vi "Interface.vi"() -> ()   [LabVIEW 2016, in "Command Interface.lvclass"]
uses:
  Command Interface.lvclass
  Universal Robot/Universal Robot.lvclass
  C:/_Code/Development/UR Dashboard Server/Classes/Application Interface/Application Interface.lvclass
  Application/Application.lvclass
  Application Interface/Application Interface.lvclass
panel:
  in  "command":u16(ring) items=["Load", "Play", "Stop", "Pause", "Quit", "Shutdown", "Running", "Robotmode", "get loaded program", "popup", "close popup", "addToLog", "IsProgramSaved", "programState", "PolyscopeVersion", "set operational mode", "clear operational mode", "power on", "power off", "brake release", "safetymode", "safetystatus", "unlock protective stop", "close safety popup", "load installation", "restart safety", "get operational mode", "is in remote control", "get serial number", "get robot model", "generate flight report", "generate support file"]
  in  "input":string
  out "inputType":string
  out "warning":string
  in  "send":bool
  out "returnStatus":string
  out "data":string
  in  "interface":refnum<class "Command Interface.lvclass">
  in  "robot":refnum<class "Universal Robot.lvclass">
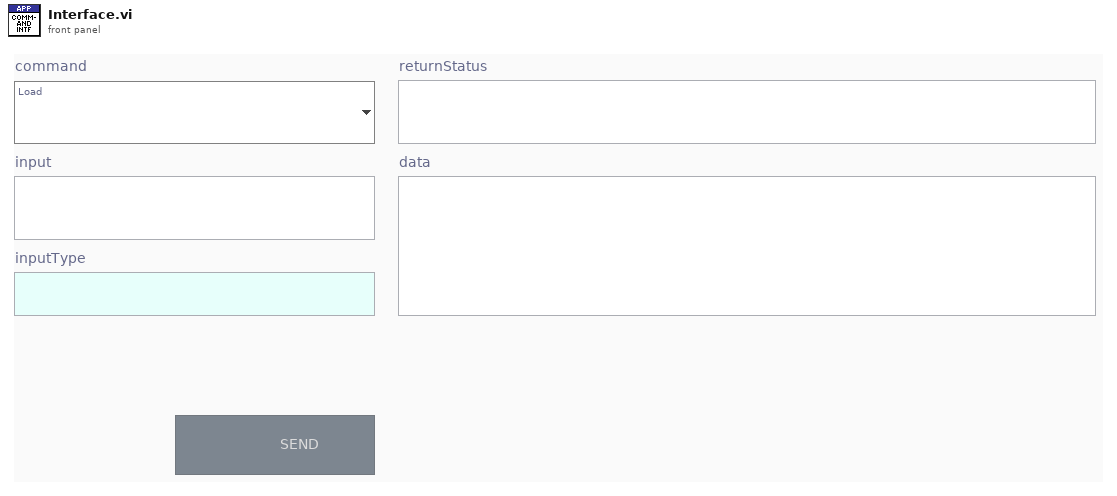
[diagram p1: front panel]
types:
  T1 = enum8{"Enabled", "Disabled", "Disabled and Grayed Out"}
  T2 = typedef "Application.lvclass/FrontPanelControls.ctl" = cluster{"General Interface":refnum<vi>, "Program Interface":refnum<vi>, "Command Interface":refnum<vi>}
  T3 = typedef "Universal Robot.lvclass/PolyScopeCommand.ctl" = cluster{"Command":string, "Input":bool, "Input Type":string, "Remote Mode Required":bool, "Min Version":T4, "Deprecated":bool}
  T4 = typedef "Universal Robot.lvclass/PolyScopeVersion.ctl" = cluster{"Major":i32, "Minor":i32, "Fix":i32, "Build":i32}
  T5 = typedef "Universal Robot.lvclass/RobotStatus.ctl" = cluster{"Robot Mode":T6, "Operational Mode":T7, "Safety Status":T8, "Remote Control":bool}
  T6 = typedef "Universal Robot.lvclass/RobotMode.ctl" = enum16{"INVALID", "NO_CONTROLLER", "DISCONNECTED", "CONFIRM_SAFETY", "BOOTING", "POWER_OFF", "POWER_ON", "IDLE", "BACKDRIVE", "RUNNING"}
  T7 = typedef "Universal Robot.lvclass/OperationalMode.ctl" = enum16{"NONE", "MANUAL", "AUTOMATIC"}
  T8 = typedef "Universal Robot.lvclass/SafetyStatus.ctl" = enum16{"INVALID", "NORMAL", "REDUCED", "PROTECTIVE_STOP", "RECOVERY", "SAFEGAURD_STOP", "SYSTEM_EMERGENCY_STOP", "ROBOT_EMERGENCY_STOP", "VIOLATION", "FAULT", "AUTOMATIC_MODE_SAFEGAURD_STOP", "SYSTEM_THREE_POSITION_ENABLING_STOP"}
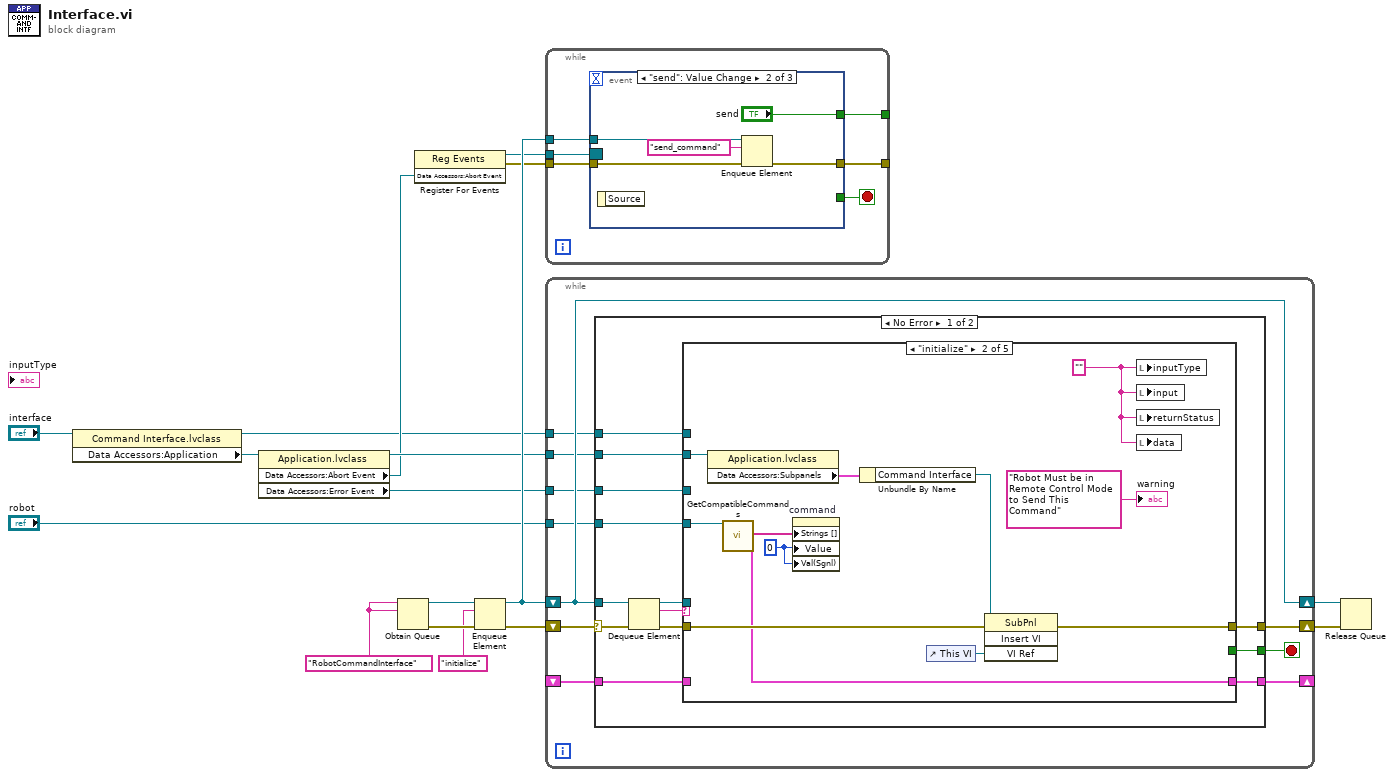
[diagram p0: block diagram]
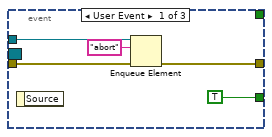
[diagram p2: hidden frame]
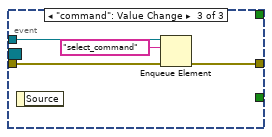
[diagram p3: hidden frame]
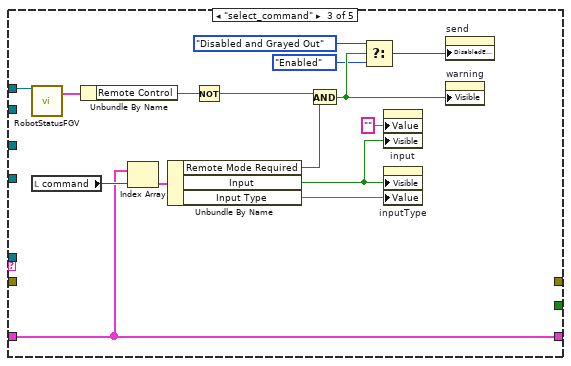
[diagram p5: hidden frame]
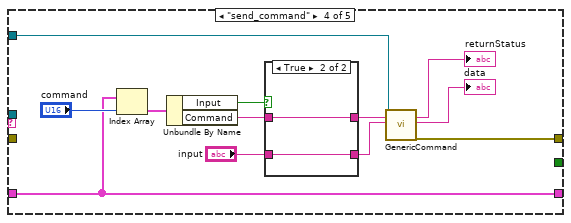
[diagram p6: hidden frame]
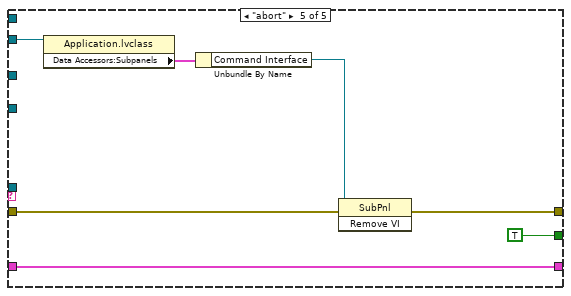
[diagram p8: hidden frame]
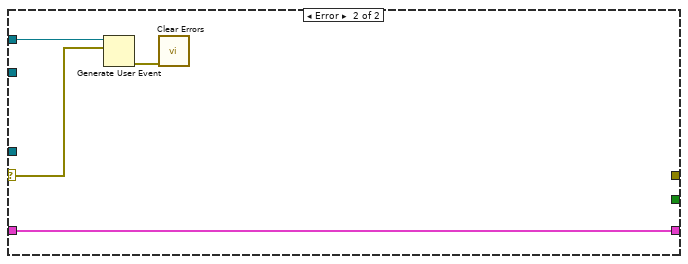
[diagram p9: hidden frame]
diagram:
  w12 = "RobotCommandInterface" ("name (unnamed)")
  n1 = property class="Command Interface.lvclass"(reference="interface") -> (reference out=w1:refnum<class "Command Interface.lvclass">, "Data Accessors:Application"=w6:refnum<class "Application.lvclass">)  [unwired: 1 in, 1 out]
  n2 = property class="Application.lvclass"(reference=w6) -> (reference out=w5:refnum<class "Application.lvclass">, "Data Accessors:Abort Event"=w4:refnum<user-event>, "Data Accessors:Error Event"=w3:refnum<user-event>)  [unwired: 1 in, 1 out]
  n3 = Obtain Queue(name (unnamed)=w12, element data type=w12) -> (queue out=w16:refnum<queue>, error out=w17:errorcluster)  [unwired: 3 in, 1 out]
  n4 = register-events(w4) -> (reference out=w8:refnum<event-registration>, error out=w9:errorcluster)  [unwired: 2 in]
  n5 = Enqueue Element(queue=w16, element="initialize", error in (no error)=w17) -> (queue out=w13:refnum<queue>, error out=w14:errorcluster)  [unwired: 1 in, 1 out]
  n6 = while {
    tunnel: w13 -> [w23]
    tunnel: w9 -> [w22]
    tunnel: w8 -> [w21]
    tunnel: [w20] -> _
    tunnel: [w18] -> _
    stop <- w19 stop-if-true
    n7 = event shown="[1] \"send\": Value Change" {
      selector: w21 -> [_ _ _]
      dyn-events: _ -> [_ _ _]
      timeout: _ -> [_ _ _]
      tunnel: w23 -> [w28 w33 w37]
      tunnel: w22 -> [w27 w32 w36]
      tunnel: [w26 w31 w35] -> w20
      tunnel: [TRUE _ _] -> w19
      tunnel: [_ "send" _] -> w18
      event User Event {
        n8 = event-data() -> ()  [unwired: 1 in, 1 out]
        n9 = Enqueue Element(queue=w28, element="abort", error in (no error)=w27) -> (error out=w26:errorcluster)  [unwired: 1 in, 2 out]
      }
      event "send": Value Change {
        n10 = event-data() -> ()  [unwired: 1 in, 1 out]
        n11 = Enqueue Element(queue=w33, element="send_command", error in (no error)=w32) -> (error out=w31:errorcluster)  [unwired: 1 in, 2 out]
      }
      event "command": Value Change {
        n12 = event-data() -> ()  [unwired: 1 in, 1 out]
        n13 = Enqueue Element(queue=w37, element="select_command", error in (no error)=w36) -> (error out=w35:errorcluster)  [unwired: 1 in, 2 out]
      }
    }
  }
  n14 = while {
    shift-right: [w45] -> w10
    shift-left: w14 -> [w47]
    shift-right: [w46] -> w11
    shift-left: w13 -> [w46]
    tunnel: w5 -> [w43]
    tunnel: "robot" -> [w42]
    shift-right: [w41] -> _
    shift-left: _ -> [w40]
    tunnel: w3 -> [w39]
    tunnel: w1 -> [w38]
    stop <- w44 stop-if-true
    n15 = case shown="No Error" w47 {
      selector: w47 -> [w59 w115]
      tunnel: w46 -> [w60 _]
      tunnel: [w55 _] -> w45
      tunnel: [w54 _] -> w44
      tunnel: w43 -> [w53 _]
      tunnel: w42 -> [w52 _]
      tunnel: [w51 w113] -> w41
      tunnel: w40 -> [w50 w113]
      tunnel: w39 -> [w49 w112]
      tunnel: w38 -> [w48 _]
      frame No Error {
        n16 = Dequeue Element(queue=w60, error in (no error)=w59) -> (queue out=w56:refnum<queue>, element=w57:string, error out=w58:errorcluster)  [unwired: 1 in, 1 out]
        n17 = case shown="\"initialize\"" w57 {
          tunnel: w58 -> [w62 w72 _ _ w110]
          tunnel: w56 -> [_ _ _ _ _]
          tunnel: [w62 w74 _ w95 w109] -> w55
          tunnel: [_ _ _ _ TRUE] -> w54
          tunnel: w53 -> [_ w67 _ _ w107]
          tunnel: w52 -> [_ w70 _ w92 _]
          tunnel: [w61 w68 w88 w100 w108] -> w51
          tunnel: w50 -> [w61 _ w88 w100 w108]
          tunnel: w49 -> [_ _ _ _ _]
          tunnel: w48 -> [_ _ w83 _ _]
          frame Default {
          }
          frame "initialize" {
            w63 = 0
            w71 = "" ("inputType")
            n18 = property class="Application.lvclass"(reference=w67) -> ("Data Accessors:Subpanels"=w66:T2)  [unwired: 1 in, 2 out]
            n19 = call-dynamic "GetCompatibleCommands.vi"("Universal Robot in"=w70) -> ("compatibleCommandList"=w69:string[], "compatibleCommands"=w68:T3[])  [unwired: 16 in, 1 out]
            n20 = property on="command" class="Ring (strict)"("Strings []"=w69, "Value"=w63, "Val(Sgnl)"=w63) -> ()  [unwired: 2 in, 2 out]
            n21 = Unbundle By Name(w66) -> ("Command Interface"=w65:refnum<vi>)
            n22 = control-ref of="This VI"() -> (w73:refnum<vi>)
            n23 = invoke class="SubPnl" method="Insert VI"(reference=w65, error in=w72, "VI Ref"=w73) -> (error out=w74:errorcluster)  [unwired: 1 in, 3 out]
            n24 = local write "inputType"(w71) -> ()
            n25 = local write "input"(w71) -> ()
            n26 = local write "returnStatus"(w71) -> ()
            n27 = local write "data"(w71) -> ()
            "warning" <- "Robot Must be in Remote Control Mode to Send This Command" ("warning")
          }
          frame "select_command" {
            n28 = call "RobotStatusFGV.vi"("Application Interface in"=w83) -> ("Robot Status out"=w82:T5)  [unwired: 16 in, 2 out]
            n29 = local read "command"() -> (w89:u16)
            n30 = Unbundle By Name(w82) -> ("Remote Control"=w80:bool)
            n31 = Index Array(array=w88, index=w89) -> (element=w87:T3)
            n32 = Unbundle By Name(w87) -> ("Remote Mode Required"=w81:bool, "Input"=w85:bool, "Input Type"=w86:string)
            n33 = Not(x=w80) -> (.not. x?=w79:bool)
            n34 = And(x=w79, y=w81) -> (x .and. y?=w78:bool)
            n35 = Select(t=T1."Disabled and Grayed Out" ("Disabled"), s=w78, f=T1."Enabled" ("Disabled")) -> (s? t:f=w75:T1)
            n36 = property on="input" class="Str"("Value"="" ("input"), "Visible"=w85) -> ()  [unwired: 2 in, 2 out]
            n37 = property on="inputType" class="Str"("Visible"=w85, "Value"=w86) -> ()  [unwired: 2 in, 2 out]
            n38 = property on="send" class="Bool"("DisabledEnum"=w75) -> ()  [unwired: 2 in, 2 out]
            n39 = property on="warning" class="Str"("Visible"=w78) -> ()  [unwired: 2 in, 2 out]
          }
          frame "send_command" {
            n40 = Index Array(array=w100, index="command") -> (element=w99:T3)
            n41 = Unbundle By Name(w99) -> ("Input"=w98:bool, "Command"=w97:string)
            n42 = case shown="True" w98 {
              tunnel: w97 -> [w102 w104]
              tunnel: [w102 w104] -> w91
              tunnel: "input" -> [_ w103]
              tunnel: [_ w103] -> w90
              frame False {
              }
              frame True {
              }
            }
            n43 = call-dynamic "GenericCommand.vi"("Universal Robot.lvclass in"=w92, "command"=w91, "data"=w90) -> ("returnStatus"=→"returnStatus":string, "data out"=→"data":string, "error out"=w95:errorcluster)  [unwired: 13 in, 1 out]
          }
          frame "abort" {
            n44 = property class="Application.lvclass"(reference=w107) -> ("Data Accessors:Subpanels"=w106:T2)  [unwired: 1 in, 2 out]
            n45 = Unbundle By Name(w106) -> ("Command Interface"=w105:refnum<vi>)
            n46 = invoke class="SubPnl" method="Remove VI"(reference=w105, error in=w110) -> (error out=w109:errorcluster)  [unwired: 1 in, 2 out]
          }
        }
      }
      frame Error {
        n47 = Generate User Event(user event=w112, event data cluster=w115) -> (error out=w114:errorcluster)  [unwired: 2 in, 1 out]
        n48 = call <vilib>:"Clear Errors.vi"("error in (no error)"=w114) -> ()  [unwired: 5 in, 2 out]
      }
    }
  }
  n49 = Release Queue(queue=w11, error in (no error)=w10) -> ()  [unwired: 1 in, 3 out]
